vi "Set Wheel Parameter by Name.vi"(8 "error in (no error)":errorcluster, 9 "parameter value":variant, 10 "parameter name":string, 11 "wheel in":refnum<class "NI_Robotics_Steering Wheel.lvclass">) -> (0 "error out":errorcluster, 1 "set?":bool, 3 "wheel out":refnum<class "NI_Robotics_Steering Wheel.lvclass">)   [LabVIEW 2017, in "NI_Robotics_Steering Wheel.lvclass"]
uses:
  <vilib>/robotics/Steering/Steering Wheel/NI_Robotics_Steering Wheel.lvclass
  <vilib>/robotics/Steering/Steering Wheel/NI_Robotics_Steering Wheel.lvclass/NI_Robotics_Steering Wheel.ctl
  <vilib>/robotics/Actuation/Motor Communication/NI_Robotics_Motor Communication.lvclass
  <vilib>/robotics/Steering/Wheel/NI_Robotics_Wheel.lvclass
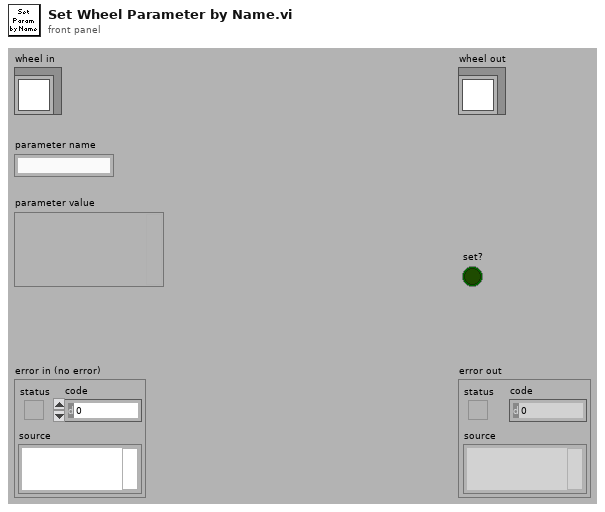
[diagram p1: front panel]
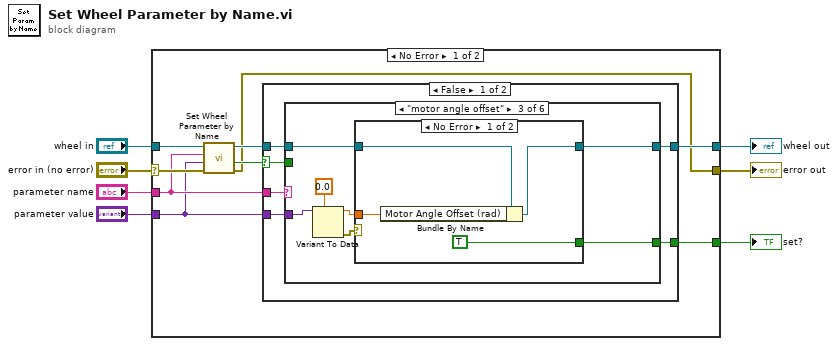
[diagram p0: block diagram]
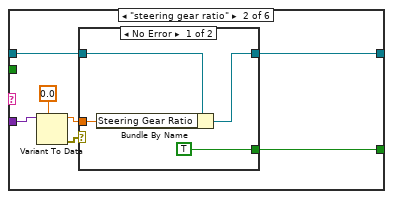
[diagram p3: hidden frame]
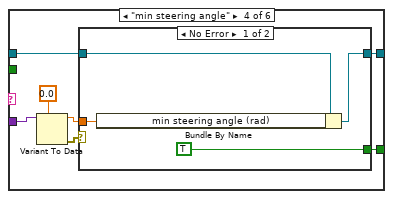
[diagram p6: hidden frame]
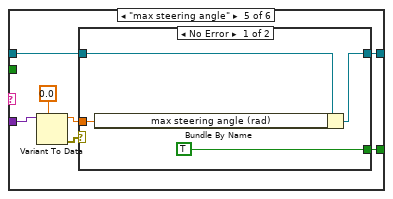
[diagram p8: hidden frame]
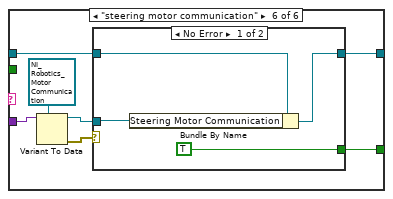
[diagram p10: hidden frame]
diagram:
  n1 = case shown="No Error" "error in (no error)" {
    selector: "error in (no error)" -> [w15 w86]
    tunnel: "parameter value" -> [w9 _]
    tunnel: "parameter name" -> [w10 _]
    tunnel: "wheel in" -> [w16 w87]
    tunnel: [w12 w87] -> w4
    tunnel: [w8 w86] -> w2
    tunnel: [w11 _] -> w1
    frame No Error {
      n2 = call-parent "Set Wheel Parameter by Name.vi"("error in (no error)"=w15, "parameter value"=w9, "parameter name"=w10, "wheel in"=w16) -> ("error out"=w8:errorcluster, "set?"=w14:bool, "wheel out"=w13:refnum<class "NI_Robotics_Steering Wheel.lvclass">)  [unwired: 5 in]
      n3 = case shown="False" w14 {
        selector: w14 -> [w19 w84]
        tunnel: w13 -> [w22 w85]
        tunnel: [w20 w85] -> w12
        tunnel: w10 -> [w21 _]
        tunnel: [w18 w84] -> w11
        tunnel: w9 -> [w17 _]
        frame False {
          n4 = case shown="\"motor angle offset\"" w21 {
            tunnel: w22 -> [w23 w30 w42 w54 w66 w78]
            tunnel: [w23 w29 w41 w53 w65 w77] -> w20
            tunnel: w19 -> [_ _ _ _ _ _]
            tunnel: [_ w24 w36 w48 w60 w73] -> w18
            tunnel: w17 -> [_ w28 w40 w52 w64 w76]
            frame Default {
            }
            frame "steering gear ratio" {
              n5 = Variant To Data(type=0.0 ("Steering Gear Ratio"), Variant=w28) -> (data=w25:dbl, error out=w26:errorcluster)  [unwired: 1 in]
              n6 = case shown="No Error" w26 {
                tunnel: w30 -> [w34 w35]
                tunnel: [w33 w35] -> w29
                tunnel: w25 -> [w32 _]
                tunnel: [TRUE _] -> w24
                frame No Error {
                  n7 = Bundle By Name(cluster=w34, "Steering Gear Ratio"=w32) -> (w33:refnum<class "NI_Robotics_Steering Wheel.lvclass">)
                }
                frame Error {
                }
              }
            }
            frame "motor angle offset" {
              n8 = Variant To Data(type=0.0 ("Steering Gear Ratio"), Variant=w40) -> (data=w37:dbl, error out=w38:errorcluster)  [unwired: 1 in]
              n9 = case shown="No Error" w38 {
                tunnel: w42 -> [w46 w47]
                tunnel: [w45 w47] -> w41
                tunnel: w37 -> [w44 _]
                tunnel: [TRUE _] -> w36
                frame No Error {
                  n10 = Bundle By Name(cluster=w46, "Motor Angle Offset (rad)"=w44) -> (w45:refnum<class "NI_Robotics_Steering Wheel.lvclass">)
                }
                frame Error {
                }
              }
            }
            frame "min steering angle" {
              n11 = Variant To Data(type=0.0 ("Steering Gear Ratio"), Variant=w52) -> (data=w49:dbl, error out=w50:errorcluster)  [unwired: 1 in]
              n12 = case shown="No Error" w50 {
                tunnel: w54 -> [w58 w59]
                tunnel: [w57 w59] -> w53
                tunnel: w49 -> [w56 _]
                tunnel: [TRUE _] -> w48
                frame No Error {
                  n13 = Bundle By Name(cluster=w58, "min steering angle (rad)"=w56) -> (w57:refnum<class "NI_Robotics_Steering Wheel.lvclass">)
                }
                frame Error {
                }
              }
            }
            frame "max steering angle" {
              n14 = Variant To Data(type=0.0 ("Steering Gear Ratio"), Variant=w64) -> (data=w61:dbl, error out=w62:errorcluster)  [unwired: 1 in]
              n15 = case shown="No Error" w62 {
                tunnel: w66 -> [w70 w71]
                tunnel: [w69 w71] -> w65
                tunnel: w61 -> [w68 _]
                tunnel: [TRUE _] -> w60
                frame No Error {
                  n16 = Bundle By Name(cluster=w70, "max steering angle (rad)"=w68) -> (w69:refnum<class "NI_Robotics_Steering Wheel.lvclass">)
                }
                frame Error {
                }
              }
            }
            frame "steering motor communication" {
              n17 = Variant To Data(type=refnum<class "NI_Robotics_Motor Communication.lvclass"> refnum ("Steering Motor Communication"), Variant=w76) -> (data=w74:refnum<class "NI_Robotics_Motor Communication.lvclass">, error out=w75:errorcluster)  [unwired: 1 in]
              n18 = case shown="No Error" w75 {
                tunnel: w78 -> [w82 w83]
                tunnel: [w81 w83] -> w77
                tunnel: w74 -> [w79 _]
                tunnel: [TRUE _] -> w73
                frame No Error {
                  n19 = Bundle By Name(cluster=w82, "Steering Motor Communication"=w79) -> (w81:refnum<class "NI_Robotics_Steering Wheel.lvclass">)
                }
                frame Error {
                }
              }
            }
          }
        }
        frame True {
        }
      }
    }
    frame Error {
    }
  }
  "error out" <- w2
  "wheel out" <- w4
  "set?" <- w1
